vi "monochromator oscillates.vi"() -> ()   [LabVIEW 2010]
panel:
  in  "Seconds to wait":dbl
  in  "Method":u16(ring) items=["round to - infinity", "round to nearest", "method 3"]
  out "actual stop wavelength":dbl
  in  "current":dbl
  in  "number of oscillates":i32
  in  "Parallel Port Address":i16=888 format="%.0x"
  in  "High wavelength":dbl
  in  "low wavelength":dbl
  in  "intializing wavelength":dbl
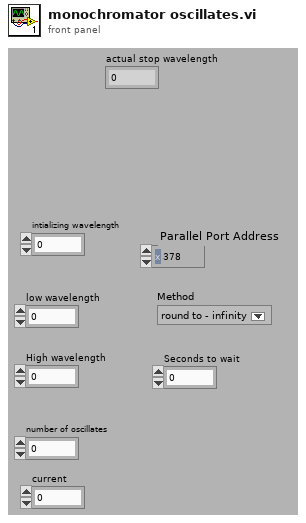
[diagram p1: front panel]
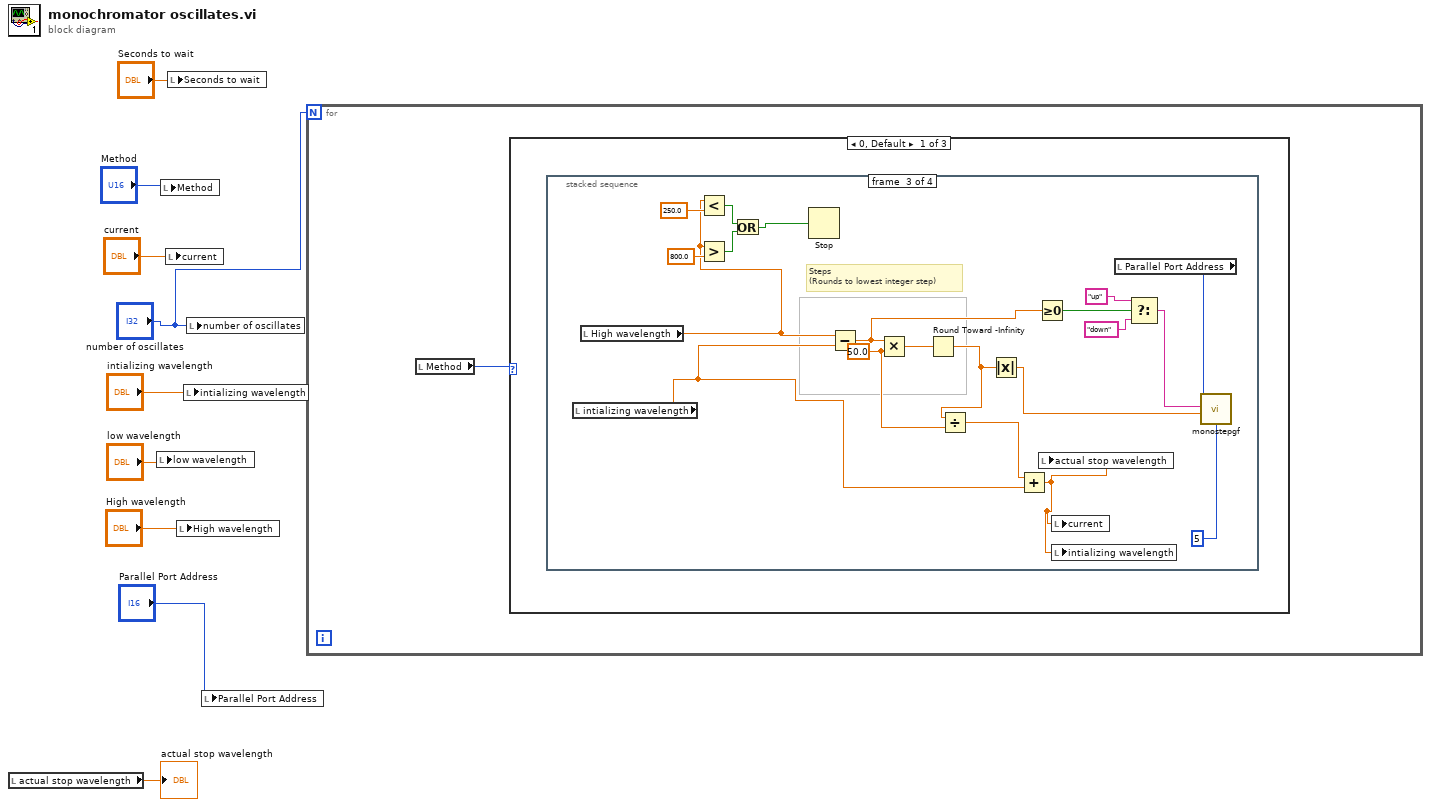
[diagram p0: block diagram]
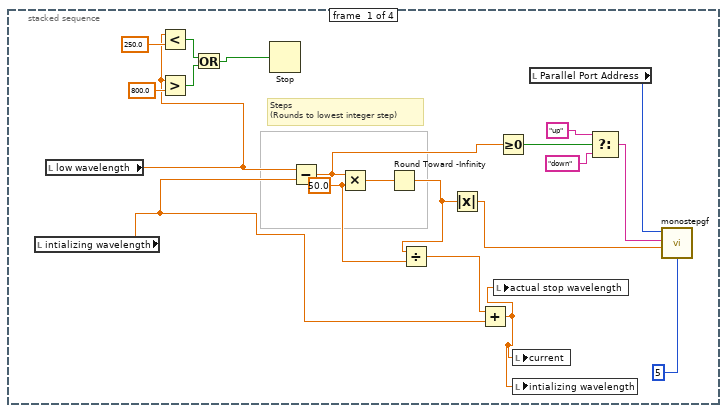
[diagram p2: hidden frame]
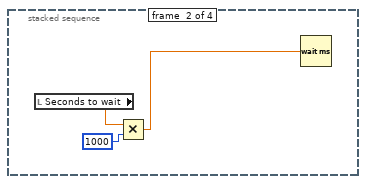
[diagram p3: hidden frame]
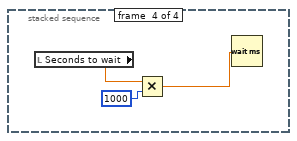
[diagram p4: hidden frame]
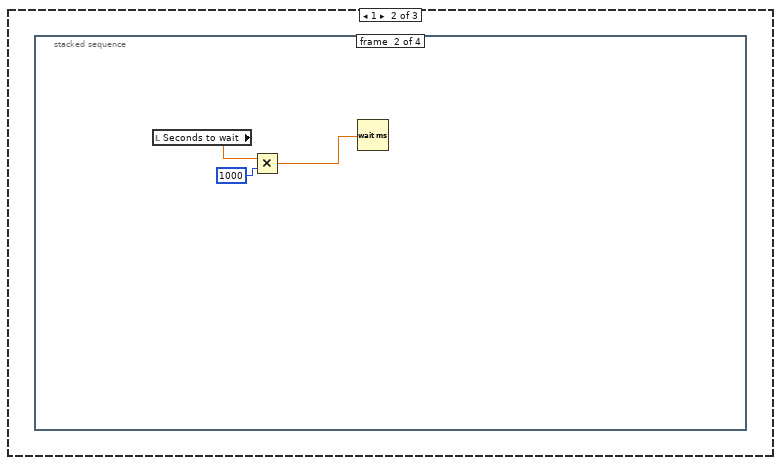
[diagram p5: hidden frame]
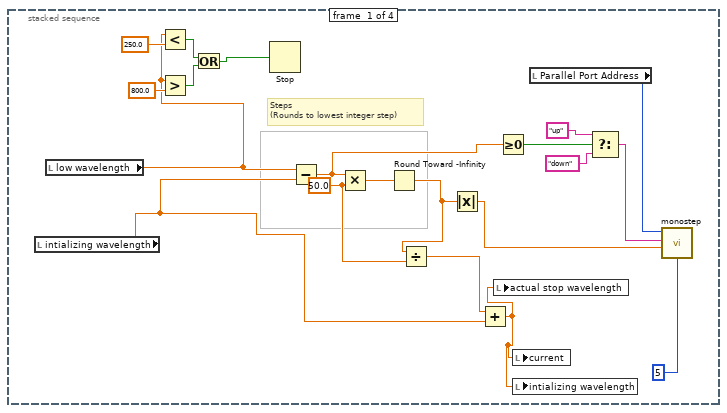
[diagram p6: hidden frame]
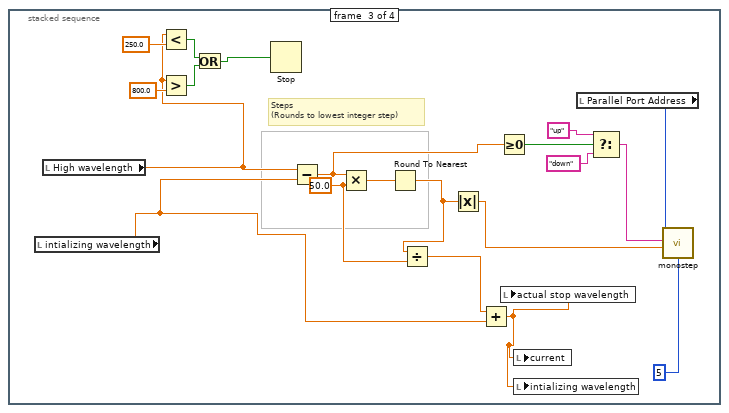
[diagram p7: hidden frame]
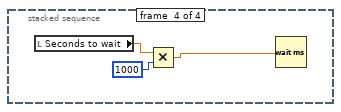
[diagram p8: hidden frame]
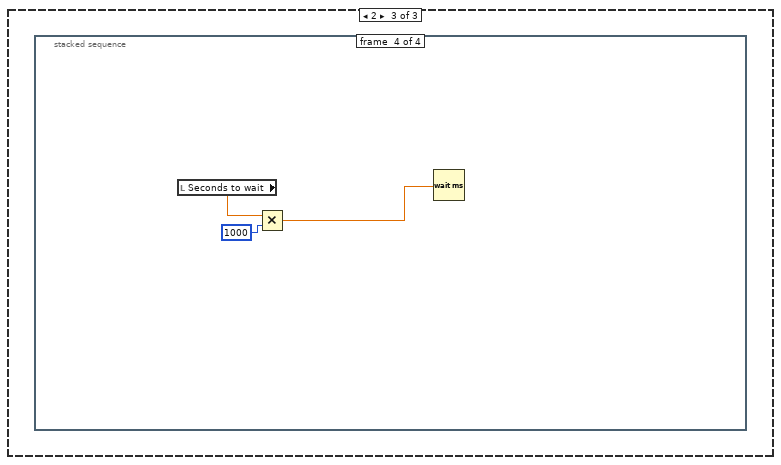
[diagram p9: hidden frame]
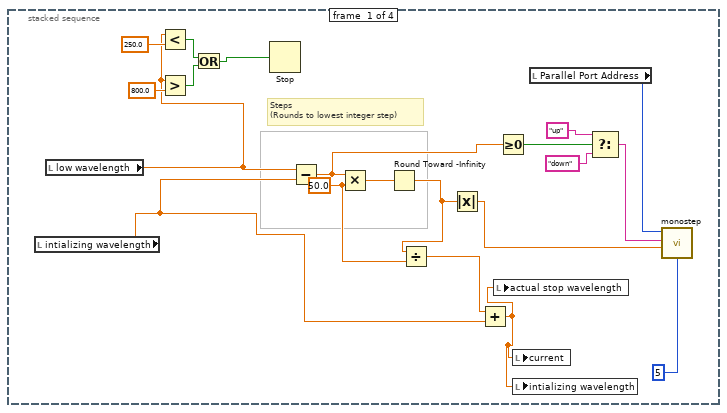
[diagram p10: hidden frame]
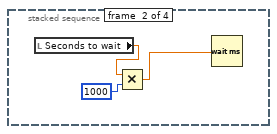
[diagram p11: hidden frame]
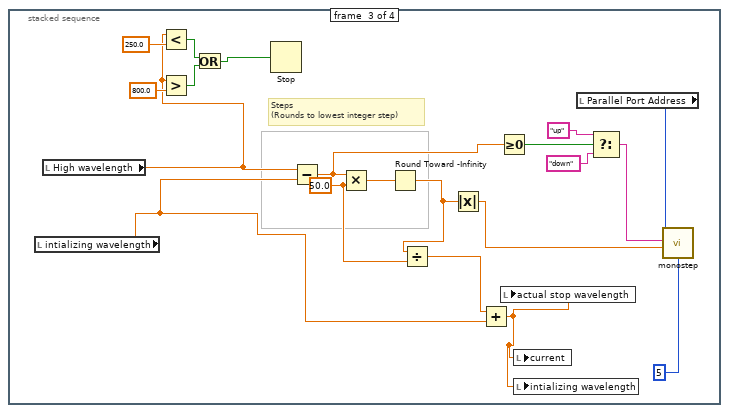
[diagram p12: hidden frame]
diagram:
  n1 = local read "actual stop wavelength"() -> (→"actual stop wavelength":dbl)
  n2 = local write "low wavelength"("low wavelength") -> ()
  n3 = local write "Method"("Method") -> ()
  n4 = local write "current"("current") -> ()
  n5 = local write "Seconds to wait"("Seconds to wait") -> ()
  n6 = local write "High wavelength"("High wavelength") -> ()
  n7 = local write "intializing wavelength"("intializing wavelength") -> ()
  n8 = local write "number of oscillates"("number of oscillates") -> ()
  n9 = local write "Parallel Port Address"("Parallel Port Address") -> ()
  n10 = for {
    N: "number of oscillates" -> [_]
    n11 = local read "Method"() -> (w10:u16)
    n12 = case shown="0, Default" w10 {
      frame 0, Default {
        n13 = stacked-sequence {
          frame #0 {
            w17 = 50.0 ("y")
            # "Steps \n(Rounds to lowest integer step)"
            n14 = local read "intializing wavelength"() -> (w13:dbl)
            n15 = local read "low wavelength"() -> (w14:dbl)
            n16 = Less?(x=w14, y=250.0) -> (x < y?=w22:bool)
            n17 = Greater?(x=w14, y=800.0) -> (0:w21:bool)
            n18 = Or(x=w22, y=w21) -> (x .or. y?=w20:bool)
            n19 = Stop(stop? (T)=w20) -> ()
            n20 = Subtract(x=w14, y=w13) -> (x-y=w29:dbl)
            n21 = Multiply(x=w29, y=w17) -> (x*y=w30:dbl)
            n22 = Round Toward -Infinity(1:w30) -> (0:w18:dbl)
            n23 = Divide(x=w18, y=w17) -> (x/y=w16:dbl)
            n24 = Absolute Value(x=w18) -> (abs(x)=w19:dbl)
            n25 = Add(x=w16, y=w13) -> (x+y=w11:dbl)
            n26 = local write "actual stop wavelength"(w11) -> ()
            n27 = Greater Or Equal To 0?(x=w29) -> (x >= 0?=w28:bool)
            n28 = local write "current"(w11) -> ()
            n29 = local write "intializing wavelength"(w11) -> ()
            n30 = local read "Parallel Port Address"() -> (w12:i16)
            n31 = Select(t="up", s=w28, f="down") -> (s? t:f=w25:string)
            n32 = call "monostepgf.vi"("Wait Between Steps(ms)"=5, "Steps"=w19, "Direction"=w25, "address"=w12) -> ()
          }
          frame #1 {
            n33 = local read "Seconds to wait"() -> (w32:dbl)
            n34 = Multiply(x=w32, y=1000) -> (x*y=w31:dbl)
            n35 = Wait (ms)(milliseconds to wait=w31) -> ()  [unwired: 1 out]
          }
          frame #2 {
            w40 = 50.0 ("y")
            # "Steps \n(Rounds to lowest integer step)"
            n36 = local read "intializing wavelength"() -> (w36:dbl)
            n37 = local read "High wavelength"() -> (w37:dbl)
            n38 = Less?(x=w37, y=250.0) -> (x < y?=w45:bool)
            n39 = Greater?(x=w37, y=800.0) -> (0:w44:bool)
            n40 = Or(x=w45, y=w44) -> (x .or. y?=w43:bool)
            n41 = Stop(stop? (T)=w43) -> ()
            n42 = Subtract(x=w37, y=w36) -> (x-y=w52:dbl)
            n43 = Multiply(x=w52, y=w40) -> (x*y=w53:dbl)
            n44 = Round Toward -Infinity(1:w53) -> (0:w41:dbl)
            n45 = Divide(x=w41, y=w40) -> (x/y=w39:dbl)
            n46 = Absolute Value(x=w41) -> (abs(x)=w42:dbl)
            n47 = Add(x=w39, y=w36) -> (x+y=w34:dbl)
            n48 = Greater Or Equal To 0?(x=w52) -> (x >= 0?=w51:bool)
            n49 = local write "actual stop wavelength"(w34) -> ()
            n50 = local write "current"(w34) -> ()
            n51 = local write "intializing wavelength"(w34) -> ()
            n52 = local read "Parallel Port Address"() -> (w35:i16)
            n53 = Select(t="up", s=w51, f="down") -> (s? t:f=w48:string)
            n54 = call "monostepgf.vi"("Wait Between Steps(ms)"=5, "Steps"=w42, "Direction"=w48, "address"=w35) -> ()
          }
          frame #3 {
            n55 = local read "Seconds to wait"() -> (w55:dbl)
            n56 = Multiply(x=w55, y=1000) -> (x*y=w54:dbl)
            n57 = Wait (ms)(milliseconds to wait=w54) -> ()  [unwired: 1 out]
          }
        }
      }
      frame 1 {
        n58 = stacked-sequence {
          frame #0 {
            w63 = 50.0 ("y")
            # "Steps \n(Rounds to lowest integer step)"
            n59 = local read "intializing wavelength"() -> (w59:dbl)
            n60 = local read "low wavelength"() -> (w60:dbl)
            n61 = Less?(x=w60, y=250.0) -> (x < y?=w68:bool)
            n62 = Greater?(x=w60, y=800.0) -> (0:w67:bool)
            n63 = Or(x=w68, y=w67) -> (x .or. y?=w66:bool)
            n64 = Stop(stop? (T)=w66) -> ()
            n65 = Subtract(x=w60, y=w59) -> (x-y=w75:dbl)
            n66 = Multiply(x=w75, y=w63) -> (x*y=w76:dbl)
            n67 = Round Toward -Infinity(1:w76) -> (0:w64:dbl)
            n68 = Divide(x=w64, y=w63) -> (x/y=w62:dbl)
            n69 = Absolute Value(x=w64) -> (abs(x)=w65:dbl)
            n70 = Add(x=w62, y=w59) -> (x+y=w57:dbl)
            n71 = local write "actual stop wavelength"(w57) -> ()
            n72 = Greater Or Equal To 0?(x=w75) -> (x >= 0?=w74:bool)
            n73 = local write "current"(w57) -> ()
            n74 = local write "intializing wavelength"(w57) -> ()
            n75 = local read "Parallel Port Address"() -> (w58:i16)
            n76 = Select(t="up", s=w74, f="down") -> (s? t:f=w71:string)
            n77 = call "monostep.vi"("Wait Between Steps(ms)"=5, "Steps"=w65, "Direction"=w71, "address"=w58) -> ()
          }
          frame #1 {
            n78 = local read "Seconds to wait"() -> (w78:dbl)
            n79 = Multiply(x=w78, y=1000) -> (x*y=w77:dbl)
            n80 = Wait (ms)(milliseconds to wait=w77) -> ()  [unwired: 1 out]
          }
          frame #2 {
            w86 = 50.0 ("y")
            # "Steps \n(Rounds to lowest integer step)"
            n81 = local read "intializing wavelength"() -> (w82:dbl)
            n82 = local read "High wavelength"() -> (w83:dbl)
            n83 = Less?(x=w83, y=250.0) -> (x < y?=w91:bool)
            n84 = Greater?(x=w83, y=800.0) -> (0:w90:bool)
            n85 = Or(x=w91, y=w90) -> (x .or. y?=w89:bool)
            n86 = Stop(stop? (T)=w89) -> ()
            n87 = Subtract(x=w83, y=w82) -> (x-y=w98:dbl)
            n88 = Multiply(x=w98, y=w86) -> (x*y=w99:dbl)
            n89 = Round To Nearest(number=w99) -> (nearest integer value=w87:dbl)
            n90 = Divide(x=w87, y=w86) -> (x/y=w85:dbl)
            n91 = Absolute Value(x=w87) -> (abs(x)=w88:dbl)
            n92 = Add(x=w85, y=w82) -> (x+y=w80:dbl)
            n93 = Greater Or Equal To 0?(x=w98) -> (x >= 0?=w97:bool)
            n94 = local write "actual stop wavelength"(w80) -> ()
            n95 = local write "current"(w80) -> ()
            n96 = local write "intializing wavelength"(w80) -> ()
            n97 = local read "Parallel Port Address"() -> (w81:i16)
            n98 = Select(t="up", s=w97, f="down") -> (s? t:f=w94:string)
            n99 = call "monostep.vi"("Wait Between Steps(ms)"=5, "Steps"=w88, "Direction"=w94, "address"=w81) -> ()
          }
          frame #3 {
            n100 = local read "Seconds to wait"() -> (w102:dbl)
            n101 = Multiply(x=w102, y=1000) -> (x*y=w100:dbl)
            n102 = Wait (ms)(milliseconds to wait=w100) -> ()  [unwired: 1 out]
          }
        }
      }
      frame 2 {
        n103 = stacked-sequence {
          frame #0 {
            w109 = 50.0 ("y")
            # "Steps \n(Rounds to lowest integer step)"
            n104 = local read "intializing wavelength"() -> (w105:dbl)
            n105 = local read "low wavelength"() -> (w106:dbl)
            n106 = Less?(x=w106, y=250.0) -> (x < y?=w114:bool)
            n107 = Greater?(x=w106, y=800.0) -> (0:w113:bool)
            n108 = Or(x=w114, y=w113) -> (x .or. y?=w112:bool)
            n109 = Stop(stop? (T)=w112) -> ()
            n110 = Subtract(x=w106, y=w105) -> (x-y=w121:dbl)
            n111 = Multiply(x=w121, y=w109) -> (x*y=w122:dbl)
            n112 = Round Toward -Infinity(1:w122) -> (0:w110:dbl)
            n113 = Divide(x=w110, y=w109) -> (x/y=w108:dbl)
            n114 = Absolute Value(x=w110) -> (abs(x)=w111:dbl)
            n115 = Add(x=w108, y=w105) -> (x+y=w103:dbl)
            n116 = local write "actual stop wavelength"(w103) -> ()
            n117 = Greater Or Equal To 0?(x=w121) -> (x >= 0?=w120:bool)
            n118 = local write "current"(w103) -> ()
            n119 = local write "intializing wavelength"(w103) -> ()
            n120 = local read "Parallel Port Address"() -> (w104:i16)
            n121 = Select(t="up", s=w120, f="down") -> (s? t:f=w117:string)
            n122 = call "monostep.vi"("Wait Between Steps(ms)"=5, "Steps"=w111, "Direction"=w117, "address"=w104) -> ()
          }
          frame #1 {
            n123 = local read "Seconds to wait"() -> (w124:dbl)
            n124 = Multiply(x=w124, y=1000) -> (x*y=w123:dbl)
            n125 = Wait (ms)(milliseconds to wait=w123) -> ()  [unwired: 1 out]
          }
          frame #2 {
            w132 = 50.0 ("y")
            # "Steps \n(Rounds to lowest integer step)"
            n126 = local read "intializing wavelength"() -> (w128:dbl)
            n127 = local read "High wavelength"() -> (w129:dbl)
            n128 = Less?(x=w129, y=250.0) -> (x < y?=w137:bool)
            n129 = Greater?(x=w129, y=800.0) -> (0:w136:bool)
            n130 = Or(x=w137, y=w136) -> (x .or. y?=w135:bool)
            n131 = Stop(stop? (T)=w135) -> ()
            n132 = Subtract(x=w129, y=w128) -> (x-y=w144:dbl)
            n133 = Multiply(x=w144, y=w132) -> (x*y=w145:dbl)
            n134 = Round Toward -Infinity(1:w145) -> (0:w133:dbl)
            n135 = Divide(x=w133, y=w132) -> (x/y=w131:dbl)
            n136 = Absolute Value(x=w133) -> (abs(x)=w134:dbl)
            n137 = Add(x=w131, y=w128) -> (x+y=w126:dbl)
            n138 = Greater Or Equal To 0?(x=w144) -> (x >= 0?=w143:bool)
            n139 = local write "actual stop wavelength"(w126) -> ()
            n140 = local write "current"(w126) -> ()
            n141 = local write "intializing wavelength"(w126) -> ()
            n142 = local read "Parallel Port Address"() -> (w127:i16)
            n143 = Select(t="up", s=w143, f="down") -> (s? t:f=w140:string)
            n144 = call "monostep.vi"("Wait Between Steps(ms)"=5, "Steps"=w134, "Direction"=w140, "address"=w127) -> ()
          }
          frame #3 {
            n145 = local read "Seconds to wait"() -> (w147:dbl)
            n146 = Multiply(x=w147, y=1000) -> (x*y=w146:dbl)
            n147 = Wait (ms)(milliseconds to wait=w146) -> ()  [unwired: 1 out]
          }
        }
      }
    }
  }
